vi "Set Variables.vi"(8 "error in":errorcluster, 11 "Data":T1) -> (0 "error out":errorcluster)   [LabVIEW 2026, in "Runtime Configuration Support Example Engine.lvlib"]
uses:
  HW Operations.ctl
  Runtime Configuration Support Example Engine.lvlib
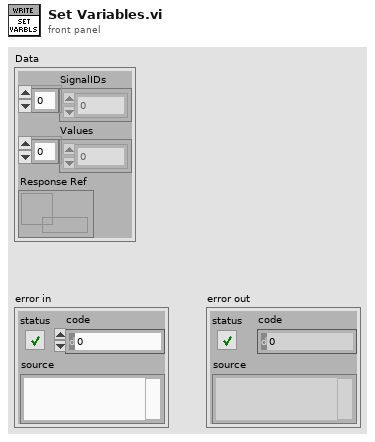
[diagram p1: front panel]
types:
  T1 = cluster{"SignalIDs":i32[], "Values":i32[], "Response Ref":refnum<queue>}
  T2 = typedef "HW Operations.ctl" = enum16{"Initialize", "Set In Val", "Get In Val", "Set Block", "Set Out Val", "Get Out Val", "Get In Array", "Get Out Array"}
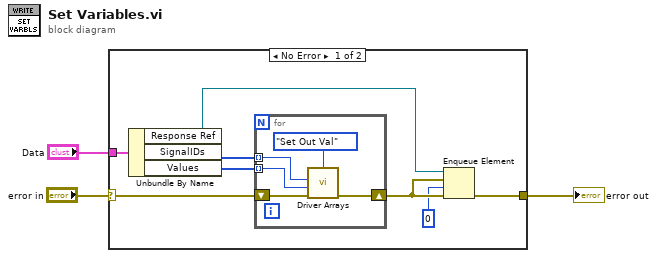
[diagram p0: block diagram]
diagram:
  n1 = case shown="No Error" "error in" {
    selector: "error in" -> [w10 w17]
    tunnel: [w9 w17] -> w3
    tunnel: "Data" -> [w8 _]
    frame No Error {
      n2 = Unbundle By Name(w8) -> ("Response Ref"=w6:refnum<queue>, "SignalIDs"=w7:i32[], "Values"=w5:i32[])
      n3 = for {
        tunnel: w7 -> [w13] mode=indexing
        shift-right: [w15] -> w11
        shift-left: w10 -> [w16]
        tunnel: w5 -> [w12] mode=indexing
        n4 = call "Driver Arrays.vi"("error in"=w16, "Value"=w12, "Index"=w13, "Curr Operation"=HW_Operations."Set Out Val") -> ("error out"=w15:errorcluster)  [unwired: 4 in, 3 out]
      }
      n5 = Enqueue Element(queue=w6, element=w11, timeout in ms (-1)=0, error in (no error)=w11) -> (error out=w9:errorcluster)  [unwired: 2 out]
    }
    frame Error {
    }
  }
  "error out" <- w3
